vi "Build Item Array Calc Child.vi"(10 "Children items":T1[](array[typedef]), 11 "Parent Item":T1) -> (3 "Concatenated items":T1[](array[typedef]))   [LabVIEW 2020, in "BlueVariantView.lvlib"]
uses:
  BlueVariantView.lvlib
  API/Typedefs/TreeData.ctl
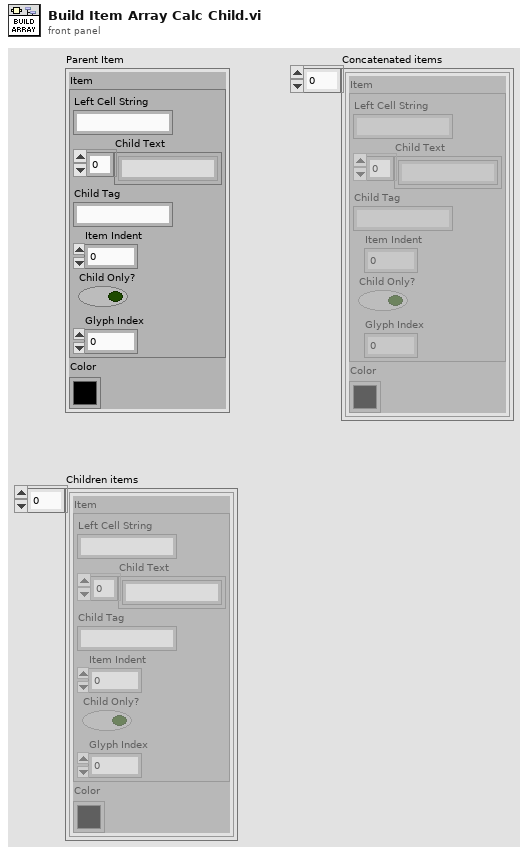
[diagram p1: front panel]
types:
  T1 = typedef "BlueVariantView.lvlib/TreeData.ctl" = cluster{"Item":cluster{"Left Cell String":string, "Child Text":string[], "Child Tag":string, "Item Indent":i32, "Child Only?":bool, "Glyph Index":i32}, "Color":u32}
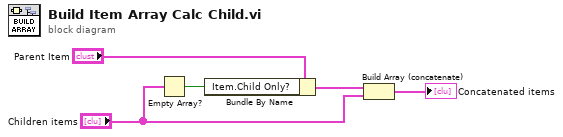
[diagram p0: block diagram]
diagram:
  n1 = Empty Array?(array="Children items") -> (empty?=w4:bool)
  n2 = Bundle By Name(cluster="Parent Item", "Item.Child Only?"=w4) -> (w3:T1)
  n3 = Build Array (concatenate)(w3, "Children items") -> (→"Concatenated items":T1[])
